vi "NI 5772 (AC) - TIS Mode Enabled (Host).vi"() -> ()   [LabVIEW 2018]
doc: "Example Description:\nThis example demonstrates how to enable Time Interleaved Sampling with the NI 5772 adapter module to achieve a sampling rate of 1.6GS/s. This example continuously acquires records of analog input data from the NI 5772 adapter module. It allows you to select an AI channel, trigger type, and record size. This VI must be compiled before it is run. \n\nVI Configuration:\nThis example uses the NI PXI-7952R as the FPGA target by default. If you are using another FPGA target, complete the following steps to configure the host VI to use a VI configured for your FPGA target:\n1. On the block diagram, right-click the Open FPGA VI Reference (NI PXI-7952R) function and select Configure Open FPGA VI Reference.\n2. Browse for a new target by clicking the Browse Project button in the Open VI section.\n3. Select the VI under the target that matches your device. Click OK to select this VI.\n4. Click OK to exit the dialog box and to apply the new selection to the FPGA VI.\n5. Save the VI.\n\nRunning the VI:\n1. Select a RIO Resource that corresponds to the FPGA device configured above.\n2. Clock Configuration: Select the desired clock source for the adapter module.\nAnalog Input: Configure the AI Channel, Record Size, and Trigger Type controls. If you are using the analog trigger type, configure the Trigger Level (V) control.\n3. Click the run arrow to run the VI.\n4. If the Trigger Type is set to Software, click the Software Trigger button to acquire a single record of data. If the Trigger Type is set to Data Edge, a record of data is acquired each time the input signal rises above the trigger level.\n\nThe Record Size, Trigger Type, and Trigger Level (V) controls can all be configured while the VI is running. \n\nNote: The AI Channel control must be configured before the VI is run.\n\nExecution Steps:s\n1. Open a session to the FPGA VI and run the VI.\n2. Wait for the adapter module to load its default configuration.\n3. Configure the NI 5772 for Time Interleaved Sampling (TIS)\n4. The Trigger type and record size for a single record acquisition are configured.\n5. Based on the trigger type, either wait for the software trigger Boolean to assert or configure the desired trigger level and arm the trigger.\n6. After the trigger is armed, a single record of data is acquired and read.\n7. Stop the VI when the stop button is pressed or when an error has occurred. \n8. Close the FPGA VI reference and display any errors."
uses:
  <vilib>/userdefined/High Color/nirio_resource_hc.ctl
  FPGA/Digitizer 5772/Controls/TIS Mode.ctl
  <vilib>/rvi/interface/RandomDataEmulation/nirviRandomDataOpen.vi
  <vilib>/rvi/interface/common/niFpgaCacheSessionInfoDynamic.vi
  <vilib>/Utility/error.llb/Error Cluster From Error Code.vi
  <vilib>/rvi/errors/niLvFpgaAdjustHostInterfaceError.vi
  <vilib>/FPGAPlugInAG/Dynamic/niLvFpga_Close_Dynamic.vi
  <vilib>/rvi/interface/nirviOpenFPGA/nirviOpenFPGA.xnode
  D:/HardwareRevamp/AcustoXv2/FPGA/Digitizer 5772/NI 5772 (AC) - TIS Mode Enabled (FPGA).vi
  <vilib>/rvi/interface/nirviReadWriteControl/nirviReadWriteControl.xnode
  <vilib>/rvi/interface/nirviMethod/nirviMethod.xnode
  <vilib>/rvi/interface/nirviCloseFPGA/nirviCloseFPGA.xnode
  NiFpgaLv.dll
  <vilib>/rvi/interface/Simulation/niFpgaSimulationCallBeginRW.vi
  <vilib>/FPGAPlugInAG/Dynamic/niLvFpga_ReadFifo_Dynamic.vi
  <vilib>/rvi/errors/niLvFpgaMergeErrorWithErrorCode.vi
panel:
  in  "Clock Source":T1(ring)=enum."Internal Clock PLL On (IoModSyncClk)"
  out "Clocking Option Configured?":bool
  in  "TIS Mode":T2=3 items=["TIS Mode (CH0 Only)"=1, "TIS Mode (CH1 Only)"=2, "Dual TIS Mode (CH0 and CH1)"=3]
  out "TIS Configured?":bool
  out "Analog Input":waveform(ext)(graph)={"t0"=timestamp(0 s since 1904-01-01), "dt"=1.25e-09, "Y"=array[2048 elements]} caption="Acquired Waveform"
  out "error out":errorcluster
  in  "stop":bool
  in  "Trigger Level (V)":dbl
  in  "Software Trigger":bool=TRUE
  in  "Record Size":u16=1024
  in  "Trigger Type":enum8{"Software", "Data Edge"}(ring)
  in  "RIO Resource":T3="PXI1Slot3"
  out "Configured?":bool
  # "Resource Configuration"
  # "AI Configuration"
  # "For instructions, select Help>>Show Context Help and move the cursor over the VI icon to display help for this VI."
  # "Interleaved Configuration"
  # "Clock Configuration"
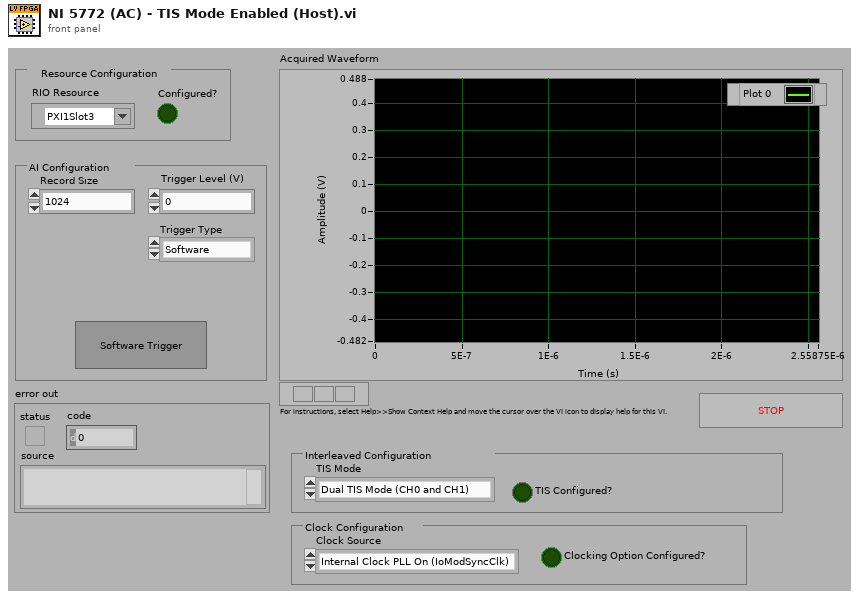
[diagram p1: front panel]
types:
  T1 = enum8{"Internal Clock PLL Off", "Internal Clock PLL On (REF IN)", "External Clock (CLK_IN)", "Internal Clock PLL On (IoModSyncClk)"}
  T2 = typedef "TIS Mode.ctl" = u16
  T3 = typedef "nirio_resource_hc.ctl" = tag
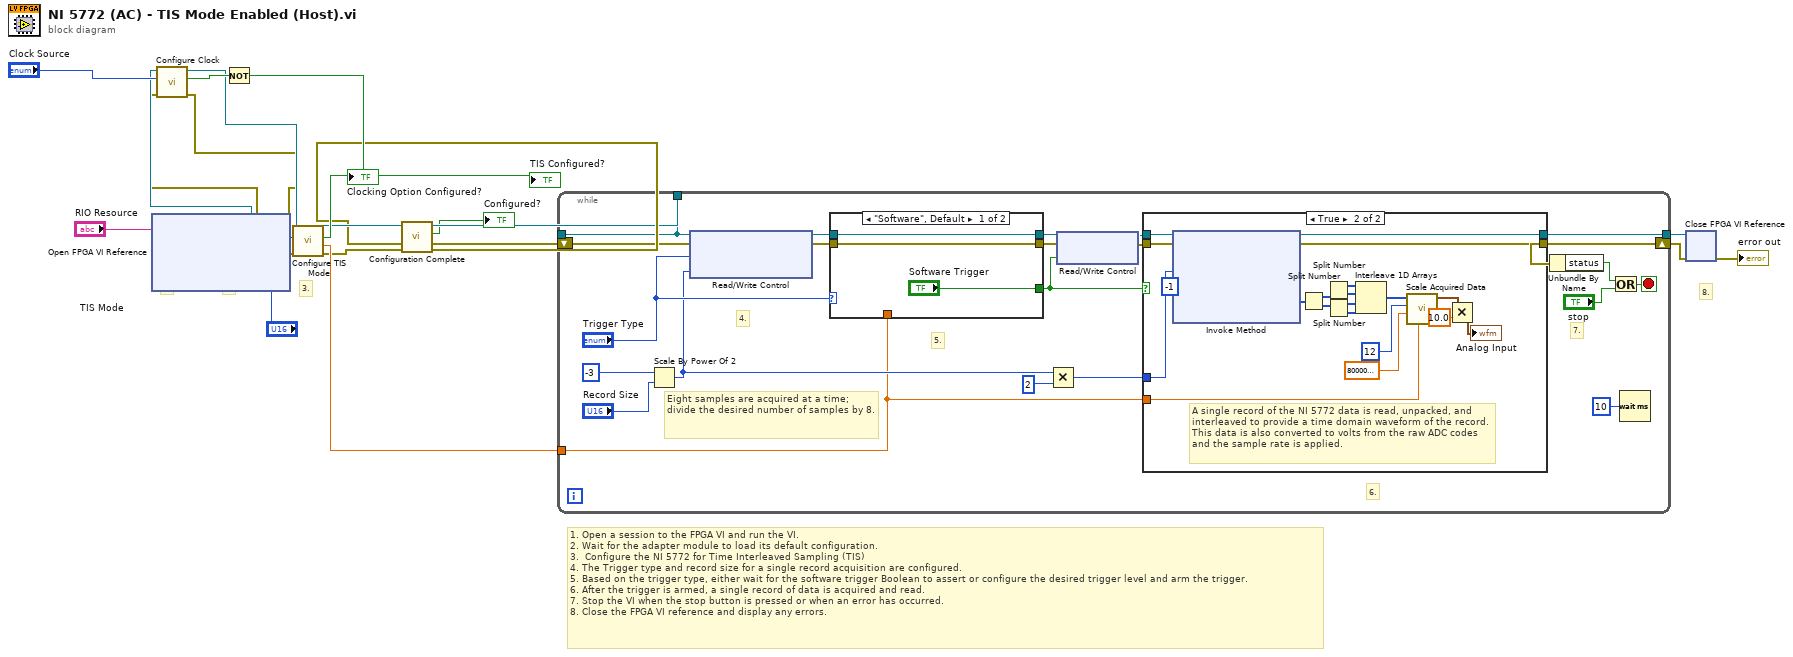
[diagram p0: block diagram]
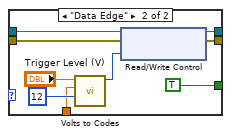
[diagram p3: hidden frame]
diagram:
  # "8."
  # "3."
  # "2."
  # "1."
  # "1. Open a session to the FPGA VI and run the VI.\n2. Wait for the adapter module to load its default configuration.\n3.  Configure the NI 5772 for Time Interleaved Sampling (TIS)\n4. The Trigger type and record size for a single record acquisition are configured.\n5. Based on the trigger type, either wait for the software trigger Boolean to assert or configure the desired trigger level and arm the trigger.\n6. After the trigger is armed, a single record of data is acquired and read.\n7. Stop the VI when the stop button is pressed or when an error has occurred.  \n8. Close the FPGA VI reference and display any errors."
  n1 = xnode "Open FPGA VI Reference"("resource name"="RIO Resource") -> ("FPGA VI Reference Out"=w7:refnum<k20>, "error out"=w6:errorcluster)  [unwired: 1 in]
  n2 = call "Configure Clock.vi"("error in"=w6, "Clock Source"="Clock Source", "FPGA VI Reference In"=w7) -> ("error out"=w8:errorcluster, "Configuration Error"=w11:bool, "FPGA VI Reference Out"=w9:refnum<k20>)  [unwired: 6 in]
  n3 = Not(x=w11) -> (.not. x?=→"Clocking Option Configured?":bool)
  n4 = call "Configure TIS Mode.vi"("error in"=w8, "TIS Mode"="TIS Mode", "FPGA VI Reference In"=w9) -> ("error out"=w4:errorcluster, "range (Vpp)"=w13:dbl, "TIS Configured?"=→"TIS Configured?":bool, "FPGA VI Reference Out"=w5:refnum<k20>)  [unwired: 5 in]
  n5 = call "Configuration Complete.vi"("error in"=w4, "FPGA VI Reference In"=w5) -> ("error out"=w3:errorcluster, "Configured?"=→"Configured?":bool, "FPGA VI Reference Out"=w2:refnum<k20>)  [unwired: 7 out]
  n6 = while {
    tunnel: [w38] -> w19
    tunnel: [w20] -> _
    shift-right: [w32] -> w17
    shift-left: w3 -> [w29]
    tunnel: w13 -> [w23]
    tunnel: w2 -> [w20]
    stop <- w28 stop-if-true
    # "7."
    # "Eight samples are acquired at a time; divide the desired number of samples by 8."
    # "6."
    # "5."
    # "4."
    n7 = Scale By Power Of 2(n=-3, x="Record Size") -> (x*2^n=w24:u16)
    n8 = xnode "Read/Write Control"("FPGA VI Reference In"=w20, "error in"=w29, "Trigger Type"="Trigger Type", "Samples Per Trigger"=w24) -> ("FPGA VI Reference Out"=w31:refnum<k20>, "error out"=w30:errorcluster)
    n9 = case shown="\"Software\", Default" "Trigger Type" {
      tunnel: w31 -> [w66 w75]
      tunnel: w30 -> [w65 w74]
      tunnel: [w66 w73] -> w37
      tunnel: [w65 w72] -> w36
      tunnel: ["Software Trigger" TRUE ("Acquire")] -> w33
      tunnel: w23 -> [_ w67]
      frame "Software", Default {
      }
      frame "Data Edge" {
        n10 = call "Volts to Codes.vi"("Number of Bits"=i16 12, "range (Vpp)"=w67, "Data In"="Trigger Level (V)") -> ("Data Out"=w68:i16)  [unwired: 8 out]
        n11 = xnode "Read/Write Control"("FPGA VI Reference In"=w75, "error in"=w74, "Trigger Level"=w68) -> ("FPGA VI Reference Out"=w73:refnum<k20>, "error out"=w72:errorcluster)
      }
    }
    n12 = Multiply(x=w24, y=u16 2) -> (x*y=w22:u16)
    n13 = xnode "Read/Write Control"("FPGA VI Reference In"=w37, "error in"=w36, "Arm Trigger"=w33) -> ("FPGA VI Reference Out"=w35:refnum<k20>, "error out"=w34:errorcluster)
    n14 = case shown="True" w33 {
      tunnel: w35 -> [w42 w63]
      tunnel: w34 -> [w43 w62]
      tunnel: [w43 w61] -> w32
      tunnel: [w42 w60] -> w38
      tunnel: w22 -> [_ w59]
      tunnel: w23 -> [_ w55]
      frame False {
      }
      frame True {
        # "A single record of the NI 5772 data is read, unpacked, and interleaved to provide a time domain waveform of the record. This data is also converted to volts from the raw ADC codes and the sample rate is applied."
        n15 = xnode "Invoke Method"("FPGA VI Reference In"=w63, "error in"=w62, "Number of Elements"=w59, "Timeout (ms)"=-1) -> ("FPGA VI Reference Out"=w60:refnum<k20>, "error out"=w61:errorcluster, "Data"=w54:u64[])  [unwired: 1 out]
        n16 = Split Number(x=w54) -> (hi(x)=w53:u32[], lo(x)=w52:u32[])
        n17 = Split Number(x=w53) -> (hi(x)=w50:u16[], lo(x)=w47:u16[])
        n18 = Split Number(x=w52) -> (hi(x)=w48:u16[], lo(x)=w49:u16[])
        n19 = Interleave 1D Arrays(w50, w47, w48, w49) -> (w51:u16[])
        n20 = call "Scale Acquired Data.vi"("range (V)"=w55, "Sample Rate"=800000000.0, "Number of Bits"=i16 12, "Data In"=w51) -> ("output waveform"=w58:waveform(ext))  [unwired: 7 out]
        n21 = Multiply(x=w58, y=10.0) -> (x*y=→"Analog Input":waveform(ext))
      }
    }
    n22 = Unbundle By Name(w32) -> ("status"=w40:bool)
    n23 = Or(x=w40, y="stop") -> (x .or. y?=w28:bool)
    n24 = Wait (ms)(milliseconds to wait=u32 10) -> ()  [unwired: 1 out]
  }
  n25 = xnode "Close FPGA VI Reference"("FPGA VI Reference In"=w19, "error in"=w17) -> ("error out"=→"error out":errorcluster)
